vi "matrix pha.vi"(8 "error in (no error)":errorcluster, 10 "n_grid":i32, 11 "field":T1) -> (0 "error out":errorcluster, 2 "matrix out 2D":dbl[][](array[numeric]), 3 "field out":T1)   [LabVIEW 2012, in "Lightpipes.lvlib"]
doc: "__declspec(dllexport) void matrix_pha(FIELD *field, double matrix[]);"
uses:
  LightPipes.lvlib
  Lightpipes.dll
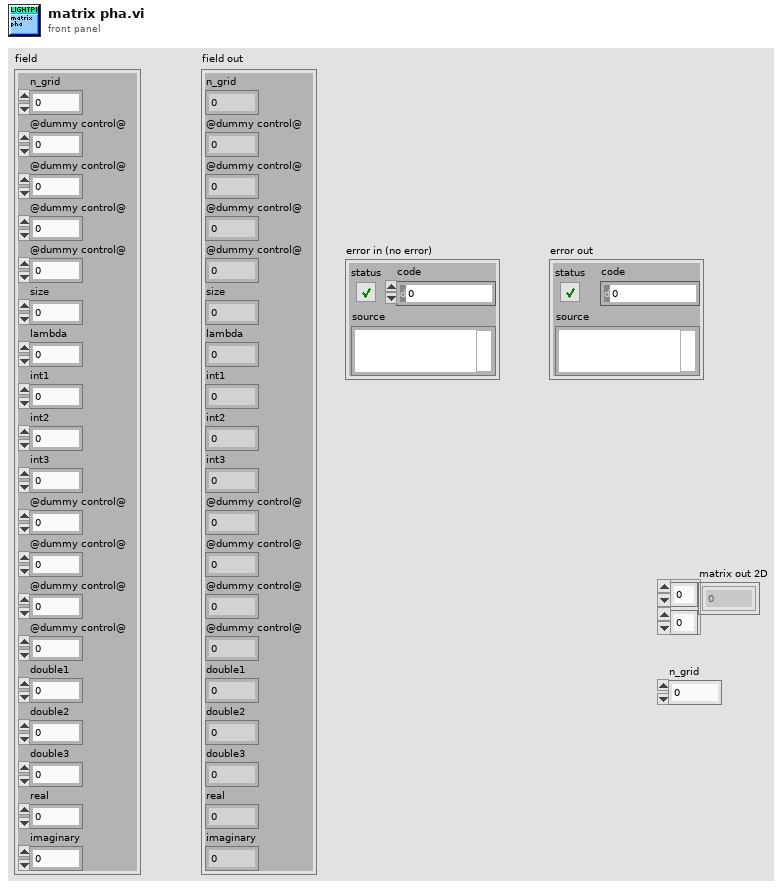
[diagram p1: front panel]
types:
  T1 = cluster{"n_grid":i32, "@dummy control@":i8, "@dummy control@":i8, "@dummy control@":i8, "@dummy control@":i8, "size":dbl, "lambda":dbl, "int1":i32, "int2":i32, "int3":i32, "@dummy control@":i8, "@dummy control@":i8, "@dummy control@":i8, "@dummy control@":i8, "double1":dbl, "double2":dbl, "double3":dbl, "real":u32, "imaginary":u32}
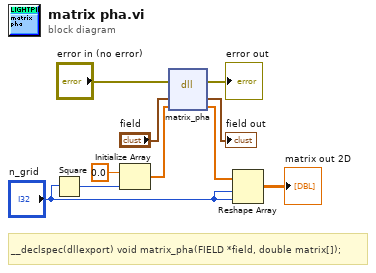
[diagram p0: block diagram]
diagram:
  # "__declspec(dllexport) void matrix_pha(FIELD *field, double matrix[]);"
  n1 = Square(x="n_grid") -> (x^2=w7:i32)
  n2 = Initialize Array(0.0 ("element"), w7) -> (w4:dbl[])
  n3 = dll-call lib="C:/Users/Tri/Documents/Lightpipes/LabView/Lightpipes.*" fn="matrix_pha"(error in="error in (no error)", "field"="field", "matrix"=w4) -> (error out=→"error out":errorcluster, "field"=→"field out":T1, "matrix"=w3:dbl[])  [unwired: 3 in, 1 out]
  n4 = Reshape Array(w3, "n_grid", "n_grid") -> (→"matrix out 2D":dbl[][])
